vi "JSONtext Path examples.vi"() -> ()   [LabVIEW 2017]
uses:
  String Subset.vi
  support/Strip Quotes and Unescape.vi
  Parse Full Path or Item Name.vi
  Find Item Locations by Path.vi
  support/Unescape JSON string.vi
  JSONtext.lvlib
panel:
  out "error out":errorcluster
  in  "Example JSON":string="[\n  {\n    \"_id\": \"596f6ff1f7404d990a1d41e3\",\n    \"index\": 0,\n    \"guid\": \"14e37125-990e-4c22-93fc-c81df96c8e52\",\n    \"isActive\": false,\n    \"balance\": \"$1,731.08\",\n    \"picture\": \"http://placehold.it/32x32\",\n    \"age\": 32,\n    \"eyeColor\": \"blue\",\n    \"name\": \"Candace Snider\",\n    \"gender\": \"female\",\n    \"company\": \"LUXURIA\",\n    \"email\": \"candacesnider@luxuria.com\",\n    \"phone\": \"+1 (836) 599-2123\",\n    \"address\": \"314 Kings Hwy, Gibsonia, New Hampshire, 6634\",\n    \"about\": \"Voluptate velit pariatur velit mollit ex Lorem ea ipsum excepteur ea ipsum. Commodo proident cillum adipisicing laboris. Laborum cupidatat et magna officia cillum fugiat excepteur ex laboris voluptate do duis. Tempor id minim id eu aliquip cupidatat excepteur cupidatat nisi elit esse duis excepteur.\\r\\n\",\n    \"registered\": \"2016-08-22T04:08:50 -01:00\",\n    \"latitude\": -9.251168,\n    \"longitude\": -117.250193,\n    \"tags\": [\n      \"officia\",\n      \"velit\",\n      \"culpa\",\n      \"consequat\",\n      \"Lorem\",\n      \"laborum\",\n      \"enim\"\n    ],\n    \"friends\": [\n      {\n        \"id\": 0,\n        \"name\": \"Mattie Chavez\"\n      },\n      {\n        \"id\": 1,\n        \"name\": \"Chan Banks\"\n      },\n      {\n        \"id\": 2,\n        \"name\": \"Angelique Coleman\"\n      }\n    ],\n    \"greeting\": \"Hello, Candace Snider! You have 4 unread messages.\",\n    \"favoriteFruit\": \"banana\"\n  },\n  {\n    \"_id\": \"596f6ff13f7d566a86aa3b8f\",\n    \"index\": 1,\n    \"guid\": \"aadae18a-2e3b-49ac-8343-e880c080933d\",\n    \"isActive\": false,\n    \"balance\": \"$2,209.91\",\n    \"picture\": \"http://placehold.it/32x32\",\n    \"age\": 30,\n    \"eyeColor\": \"brown\",\n    \"name\": \"Cummings Strickland\",\n    \"gender\": \"male\",\n    \"company\": \"LEXICONDO\",\n    \"email\": \"cummingsstrickland@lexicondo.com\",\n    \"phone\": \"+1 (865) 427-2802\",\n    \"address\": \"461 Bragg Street, Caron, Idaho, 3172\",\n    \"about\": \"Nisi aliquip ad incididunt minim. Ea et consectetur proident officia minim exercitation sunt elit commodo. Labore nulla qui do in sunt deserunt. Duis est consequat proident elit deserunt.\\r\\n\",\n    \"registered\": \"2016-12-30T12:36:16 -00:00\",\n    \"latitude\": 70.104709,\n    \"longitude\": 61.977379,\n    \"tags\": [\n      \"tempor\",\n      \"adipisicing\",\n      \"nisi\",\n      \"cupidatat\",\n      \"deserunt\",\n      \"elit\",\n      \"laborum\"\n    ],\n    \"friends\": [\n      {\n        \"id\": 0,\n        \"name\": \"Mccarty Hunt\"\n      },\n      {\n        \"id\": 1,\n        \"name\": \"Huffman Baxter\"\n      },\n      {\n        \"id\": 2,\n        \"name\": \"Eloise Kane\"\n      }\n    ],\n    \"greeting\": \"Hello, Cummings Strickland! You have 1 unread messages.\",\n    \"favoriteFruit\": \"apple\"\n  },\n  {\n    \"_id\": \"596f6ff1f5986c4ecc6415fc\",\n    \"index\": 2,\n    \"guid\": \"9c957bfb-4fa8-4bd4-a41e-af6cc60c14a3\",\n    \"isActive\": false,\n    \"balance\": \"$3,475.09\",\n    \"picture\": \"http://placehold.it/32x32\",\n    \"age\": 35,\n    \"eyeColor\": \"blue\",\n    \"name\": \"Decker Hendrix\",\n    \"gender\": \"male\",\n    \"company\": \"GALLAXIA\",\n    \"email\": \"deckerhendrix@gallaxia.com\",\n    \"phone\": \"+1 (869) 561-3450\",\n    \"address\": \"205 Irving Street, Bradenville, Rhode Island, 7175\",\n    \"about\": \"Occaecat mollit veniam qui minim fugiat sint. Qui consequat labore in in voluptate voluptate adipisicing consequat exercitation. Nostrud quis sint amet velit fugiat non ad adipisicing deserunt aliqua aliquip. Exercitation sint do eu ut laboris nostrud. Adipisicing duis sunt dolor culpa officia cupidatat nostrud cillum ea fugiat laborum adipisicing exercitation. Ad mollit eiusmod quis nisi magna cillum enim et. Fugiat pariatur esse ullamco est dolore velit magna fugiat ad culpa.\\r\\n\",\n    \"registered\": \"2015-04-06T03:36:15 -01:00\",\n    \"latitude\": 51.47993,\n    \"longitude\": -166.022245,\n    \"tags\": [\n      \"amet\",\n      \"eiusmod\",\n      \"est\",\n      \"pariatur\",\n      \"labore\",\n      \"est\",\n      \"veniam\"\n    ],\n    \"friends\": [\n      {\n        \"id\": 0,\n        \"name\": \"Chase Terrell\"\n      },\n      {\n        \"id\": 1,\n        \"name\": \"Carrie Spencer\"\n      },\n      {\n        \"id\": 2,\n        \"name\": \"Cathryn Hyde\"\n      }\n    ],\n    \"greeting\": \"Hello, Decker Hendrix! You have 8 unread messages.\",\n    \"favoriteFruit\": \"strawberry\"\n  }\n]"
  out "Table Control":string[][](table)
  in  "$Path examples (Please select)":string(combo)="$[*].friends[*].name"
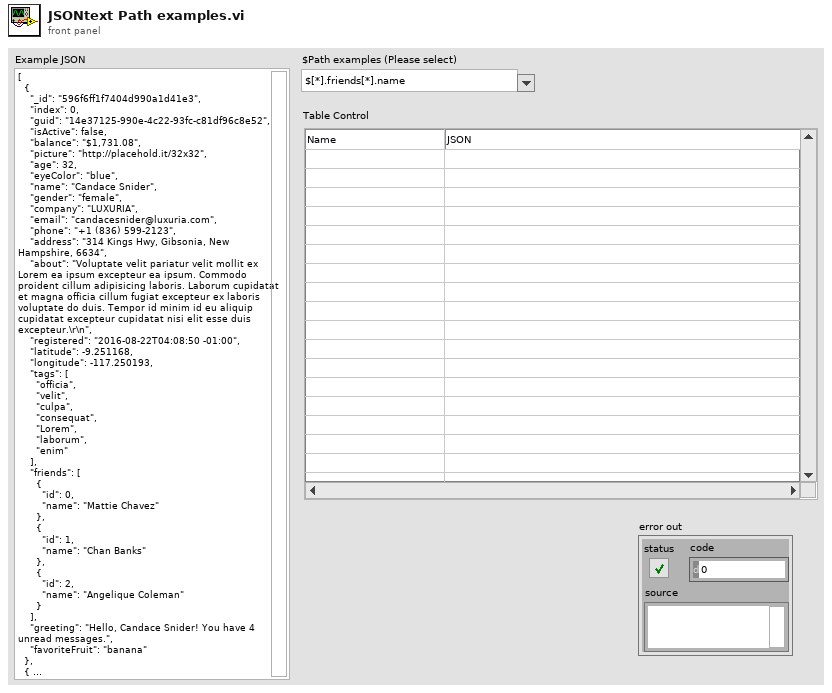
[diagram p1: front panel]
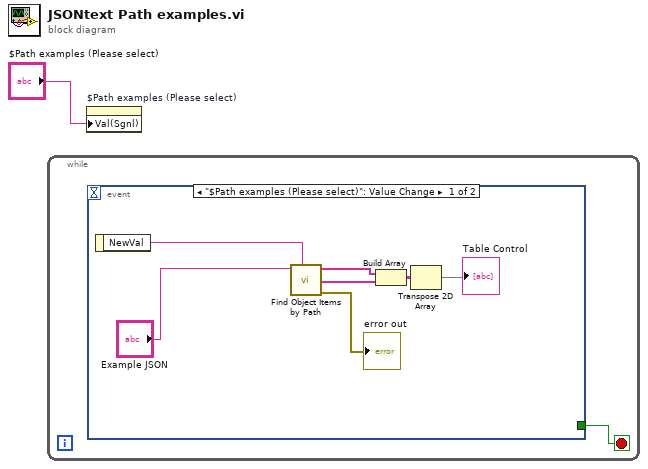
[diagram p0: block diagram]
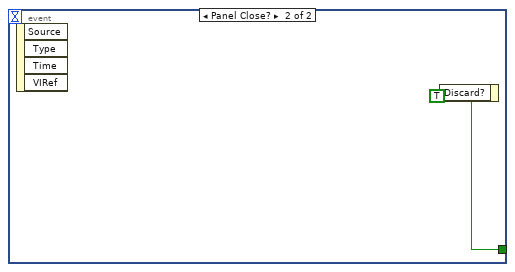
[diagram p2: hidden frame]
diagram:
  n1 = while {
    stop <- w2 stop-if-true
    n2 = event shown="[0] \"$Path examples (Please select)\": Value Change" {
      selector: _ -> [_ _]
      dyn-events: _ -> [_ _]
      timeout: _ -> [_ _]
      tunnel: [_ w10] -> w2
      event "$Path examples (Please select)": Value Change {
        n3 = event-data() -> ("NewVal"=w9:string)  [unwired: 1 in]
        n4 = call "Find Object Items by Path.vi"("$Path or Item Name"=w9, "JSON"="Example JSON") -> ("error out"=→"error out":errorcluster, "<JSON>Items"=w7:string[], "Names"=w8:string[])  [unwired: 6 in, 1 out]
        n5 = Build Array(w8, w7) -> (w6:string[][])
        n6 = Transpose 2D Array(2D array=w6) -> (transposed array=→"Table Control":string[][])
      }
      event Panel Close? {
        w10 = TRUE
        n7 = event-data() -> ()  [unwired: 1 in, 4 out]
        n8 = event-data("Discard?"=w10) -> ()  [unwired: 1 in, 1 out]
      }
    }
  }
  n9 = property on="$Path examples (Please select)" class="CmbBox"("Val(Sgnl)"="$Path examples (Please select)") -> ()  [unwired: 2 in, 2 out]
